vi "Test Unit.vi"() -> ()   [LabVIEW 2013]
uses:
  FGV Laser/Action Laser.ctl
  FGV Laser/FGV Laser Data.ctl
panel:
  in  "Read Visa":bool
  in  "Read Count":u32=10000
  out "Power Get":dbl
  in  "Power Set":dbl
  in  "Power Get":bool
  in  "Power Set":bool
  in  "Laser OFF":bool
  out "Status":string
  in  "VISA resource name out":refnum<visa-resource-name>
  in  "Laser ON":bool
  in  "stop":bool
  in  "connect":bool
  out "error out":errorcluster
  in  "Init":bool
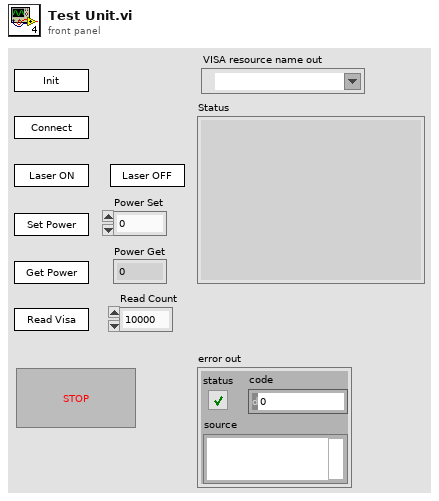
[diagram p1: front panel]
types:
  T1 = typedef "FGV Laser Data.ctl" = cluster{"ONLINE":bool, "Power":dbl, "PulsePicker":dbl, "VISA resource name out":refnum<visa-resource-name>, "Time Out":dbl, "Status":string, "Read Count":u32, "On/OFF":bool}
  T2 = typedef "Action Laser.ctl" = enum16{"Initialize", "Connect", "Disconnect", "Set Power", "Get Power", "Set Pulse Picker", "Get Pulse Picker", "Laser ON", "Laser OFF", "Read Visa"}
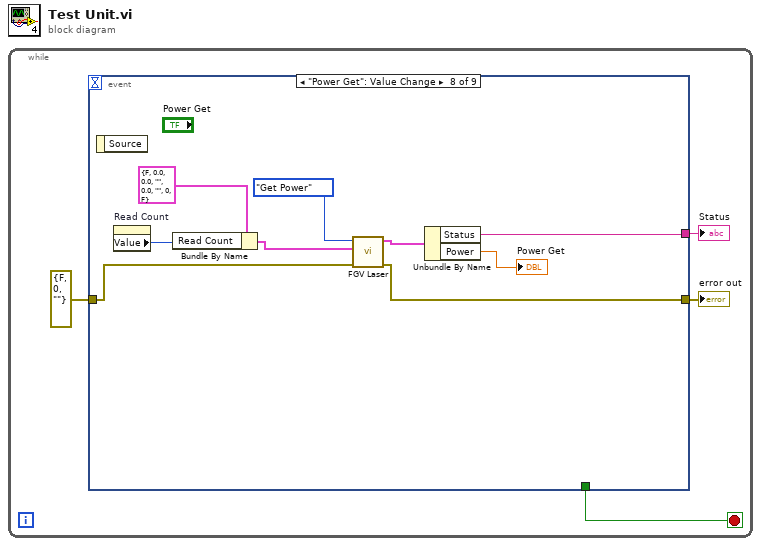
[diagram p0: block diagram]
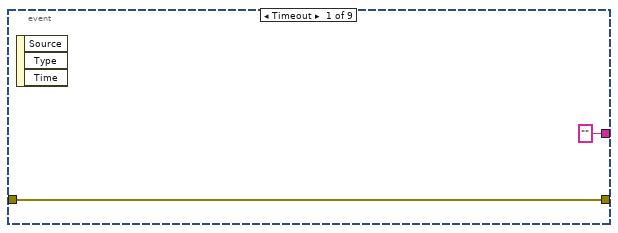
[diagram p2: hidden frame]
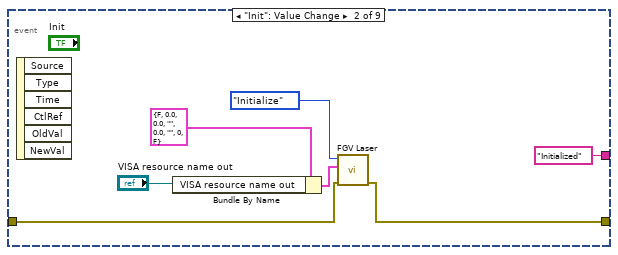
[diagram p3: hidden frame]
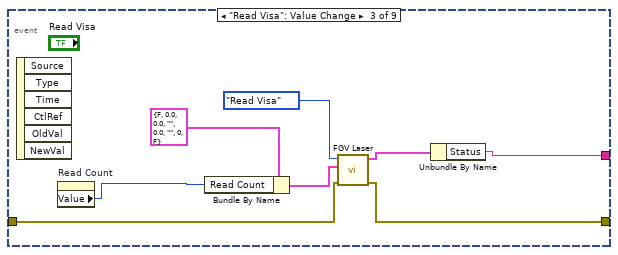
[diagram p4: hidden frame]
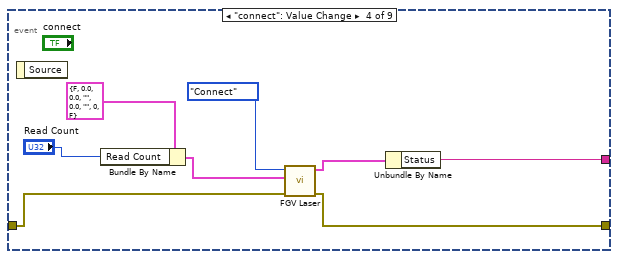
[diagram p5: hidden frame]
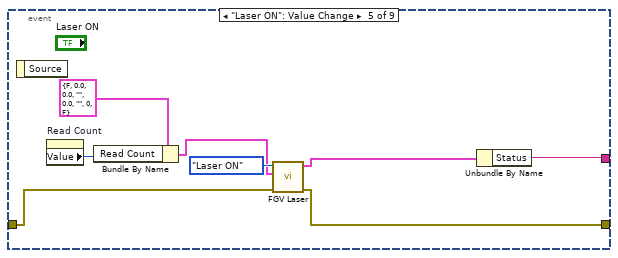
[diagram p6: hidden frame]
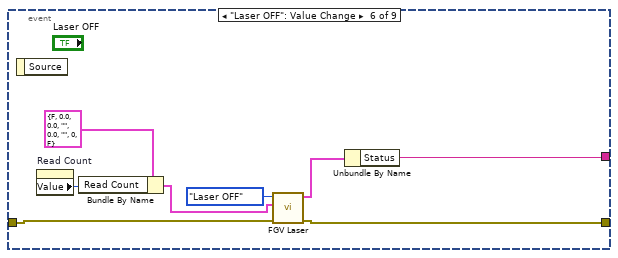
[diagram p7: hidden frame]
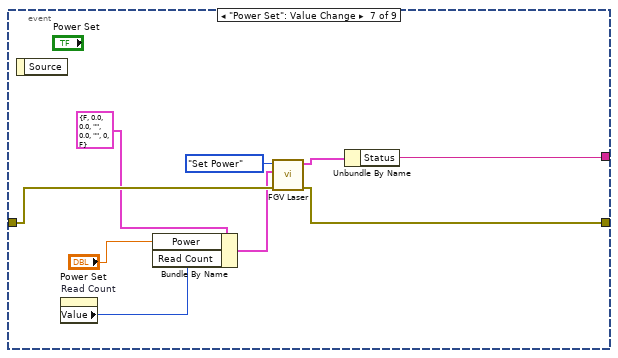
[diagram p8: hidden frame]
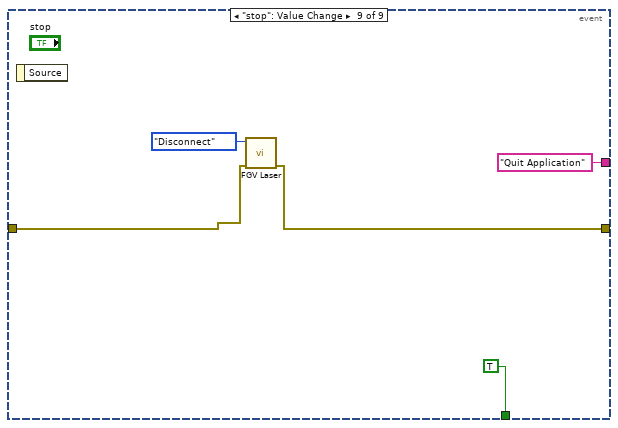
[diagram p9: hidden frame]
diagram:
  n1 = while {
    stop <- w2 stop-if-true
    n2 = event shown="[7] \"Power Get\": Value Change" {
      selector: _ -> [_ _ _ _ _ _ _ _ _]
      dyn-events: _ -> [_ _ _ _ _ _ _ _ _]
      timeout: _ -> [_ _ _ _ _ _ _ _ _]
      tunnel: errorcluster {"status"=FALSE, "code"=0, "source"=""} ("error in (no error)") -> [w6 w12 w20 w28 w35 w43 w52 w59 w65]
      tunnel: [w6 w13 w21 w27 w36 w44 w53 w62 w64] -> w3
      tunnel: [_ _ _ _ _ _ _ _ TRUE] -> w2
      tunnel: ["" ("Status") "Initialized" ("Status") w14 w25 w33 w41 w50 w60 "Quit Application" ("Status")] -> w1
      event Timeout {
        n3 = event-data() -> ()  [unwired: 1 in, 3 out]
      }
      event "Init": Value Change {
        n4 = event-data() -> ()  [unwired: 1 in, 6 out]
        n5 = Bundle By Name(cluster=T1 {"ONLINE"=FALSE, "Power"=0.0, "PulsePicker"=0.0, "VISA resource name out"="", "Time Out"=0.0, "Status"="", "Read Count"=0, "On/OFF"=FALSE} ("FGV Laser Data In"), "VISA resource name out"="VISA resource name out") -> (w9:T1)
        n6 = call "FGV Laser.vi"("error in (no error)"=w12, "FGV Laser Data In"=w9, "Action"=Action_Laser."Initialize") -> ("error out"=w13:errorcluster)  [unwired: 7 in, 1 out]
      }
      event "Read Visa": Value Change {
        n7 = event-data() -> ()  [unwired: 1 in, 6 out]
        n8 = property on="Read Count" class="DigNum (strict)"() -> ("Value"=w16:u32)  [unwired: 2 in, 2 out]
        n9 = Bundle By Name(cluster=T1 {"ONLINE"=FALSE, "Power"=0.0, "PulsePicker"=0.0, "VISA resource name out"="", "Time Out"=0.0, "Status"="", "Read Count"=0, "On/OFF"=FALSE} ("FGV Laser Data In"), "Read Count"=w16) -> (w17:T1)
        n10 = call "FGV Laser.vi"("error in (no error)"=w20, "FGV Laser Data In"=w17, "Action"=Action_Laser."Read Visa") -> ("error out"=w21:errorcluster, "FGV Laser Data Out"=w15:T1)  [unwired: 7 in]
        n11 = Unbundle By Name(w15) -> ("Status"=w14:string)
      }
      event "connect": Value Change {
        n12 = event-data() -> ()  [unwired: 1 in, 1 out]
        n13 = Bundle By Name(cluster=T1 {"ONLINE"=FALSE, "Power"=0.0, "PulsePicker"=0.0, "VISA resource name out"="", "Time Out"=0.0, "Status"="", "Read Count"=0, "On/OFF"=FALSE} ("FGV Laser Data In"), "Read Count"="Read Count") -> (w23:T1)
        n14 = call "FGV Laser.vi"("error in (no error)"=w28, "FGV Laser Data In"=w23, "Action"=Action_Laser."Connect") -> ("error out"=w27:errorcluster, "FGV Laser Data Out"=w26:T1)  [unwired: 7 in]
        n15 = Unbundle By Name(w26) -> ("Status"=w25:string)
      }
      event "Laser ON": Value Change {
        n16 = event-data() -> ()  [unwired: 1 in, 1 out]
        n17 = property on="Read Count" class="DigNum (strict)"() -> ("Value"=w30:u32)  [unwired: 2 in, 2 out]
        n18 = Bundle By Name(cluster=T1 {"ONLINE"=FALSE, "Power"=0.0, "PulsePicker"=0.0, "VISA resource name out"="", "Time Out"=0.0, "Status"="", "Read Count"=0, "On/OFF"=FALSE} ("FGV Laser Data In"), "Read Count"=w30) -> (w31:T1)
        n19 = call "FGV Laser.vi"("error in (no error)"=w35, "FGV Laser Data In"=w31, "Action"=Action_Laser."Laser ON") -> ("error out"=w36:errorcluster, "FGV Laser Data Out"=w34:T1)  [unwired: 7 in]
        n20 = Unbundle By Name(w34) -> ("Status"=w33:string)
      }
      event "Laser OFF": Value Change {
        n21 = event-data() -> ()  [unwired: 1 in, 1 out]
        n22 = property on="Read Count" class="DigNum (strict)"() -> ("Value"=w38:u32)  [unwired: 2 in, 2 out]
        n23 = Bundle By Name(cluster=T1 {"ONLINE"=FALSE, "Power"=0.0, "PulsePicker"=0.0, "VISA resource name out"="", "Time Out"=0.0, "Status"="", "Read Count"=0, "On/OFF"=FALSE} ("FGV Laser Data In"), "Read Count"=w38) -> (w39:T1)
        n24 = call "FGV Laser.vi"("error in (no error)"=w43, "FGV Laser Data In"=w39, "Action"=Action_Laser."Laser OFF") -> ("error out"=w44:errorcluster, "FGV Laser Data Out"=w42:T1)  [unwired: 7 in]
        n25 = Unbundle By Name(w42) -> ("Status"=w41:string)
      }
      event "Power Set": Value Change {
        n26 = event-data() -> ()  [unwired: 1 in, 1 out]
        n27 = property on="Read Count" class="DigNum (strict)"() -> ("Value"=w46:u32)  [unwired: 2 in, 2 out]
        n28 = Bundle By Name(cluster=T1 {"ONLINE"=FALSE, "Power"=0.0, "PulsePicker"=0.0, "VISA resource name out"="", "Time Out"=0.0, "Status"="", "Read Count"=0, "On/OFF"=FALSE} ("FGV Laser Data In"), "Power"="Power Set", "Read Count"=w46) -> (w47:T1)
        n29 = call "FGV Laser.vi"("error in (no error)"=w52, "FGV Laser Data In"=w47, "Action"=Action_Laser."Set Power") -> ("error out"=w53:errorcluster, "FGV Laser Data Out"=w51:T1)  [unwired: 7 in]
        n30 = Unbundle By Name(w51) -> ("Status"=w50:string)
      }
      event "Power Get": Value Change {
        n31 = event-data() -> ()  [unwired: 1 in, 1 out]
        n32 = property on="Read Count" class="DigNum (strict)"() -> ("Value"=w55:u32)  [unwired: 2 in, 2 out]
        n33 = Bundle By Name(cluster=T1 {"ONLINE"=FALSE, "Power"=0.0, "PulsePicker"=0.0, "VISA resource name out"="", "Time Out"=0.0, "Status"="", "Read Count"=0, "On/OFF"=FALSE} ("FGV Laser Data In"), "Read Count"=w55) -> (w56:T1)
        n34 = call "FGV Laser.vi"("error in (no error)"=w59, "FGV Laser Data In"=w56, "Action"=Action_Laser."Get Power") -> ("error out"=w62:errorcluster, "FGV Laser Data Out"=w61:T1)  [unwired: 7 in]
        n35 = Unbundle By Name(w61) -> ("Status"=w60:string, "Power"=→"Power Get":dbl)
      }
      event "stop": Value Change {
        n36 = event-data() -> ()  [unwired: 1 in, 1 out]
        n37 = call "FGV Laser.vi"("error in (no error)"=w65, "Action"=Action_Laser."Disconnect") -> ("error out"=w64:errorcluster)  [unwired: 8 in, 1 out]
      }
    }
    "error out" <- w3
    "Status" <- w1
  }
